vi "Apply Lowpass Filter.vi"(6 "state info in":T2 {"y(n-2) state" format="%.2f"; "x(n-2) state" format="%.2f"; "y(n-1) state" format="%.2f"; "x(n-1) state" format="%.2f"}, 7 "reset":bool=TRUE, 9 "filter coefficients":cluster{"beta":dbl, "gamma":dbl, "alpha":dbl} {"alpha" format="%.2f"; "gamma" format="%.2f"; "beta" format="%.2f"}, 10 "Conversion Op":T1, 11 "Input stream":waveform(sgl)={"t0"=timestamp(0 s since 1904-01-01), "dt"=0.0, "Y"=[]}) -> (3 "filtered signal":waveform(sgl), 4 "state info out":T2 {"y(n-2) state" format="%.2f"; "x(n-2) state" format="%.2f"; "y(n-1) state" format="%.2f"; "x(n-1) state" format="%.2f"})   [LabVIEW 2017, in "VibrationAnalysisFunctions.lvlib"]
uses:
  <vilib>/addons/InsightCM/Utilities/Analysis/Vibration/VibrationAnalysisFunctions.lvlib
  <vilib>/addons/InsightCM/Utilities/Analysis/Shared/controls/ConversionOp.ctl
  <vilib>/addons/InsightCM/Utilities/Analysis/Shared/AnalysisHelper.lvlib
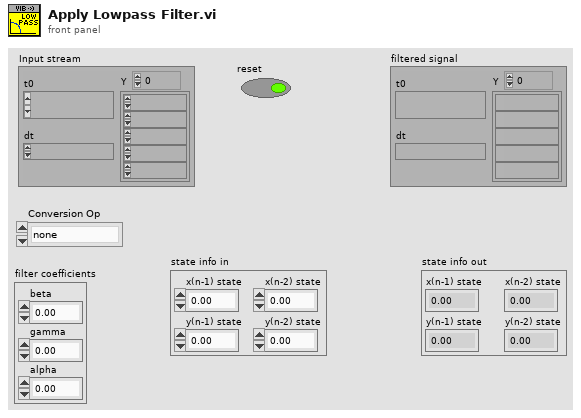
[diagram p1: front panel]
types:
  T1 = typedef "AnalysisHelper.lvlib/ConversionOp.ctl" = enum16{"none", "singleInt", "doubleInt", "singleDiff", "doubleDiff"}
  T2 = cluster{"x(n-1) state":dbl, "y(n-1) state":dbl, "x(n-2) state":dbl, "y(n-2) state":dbl}
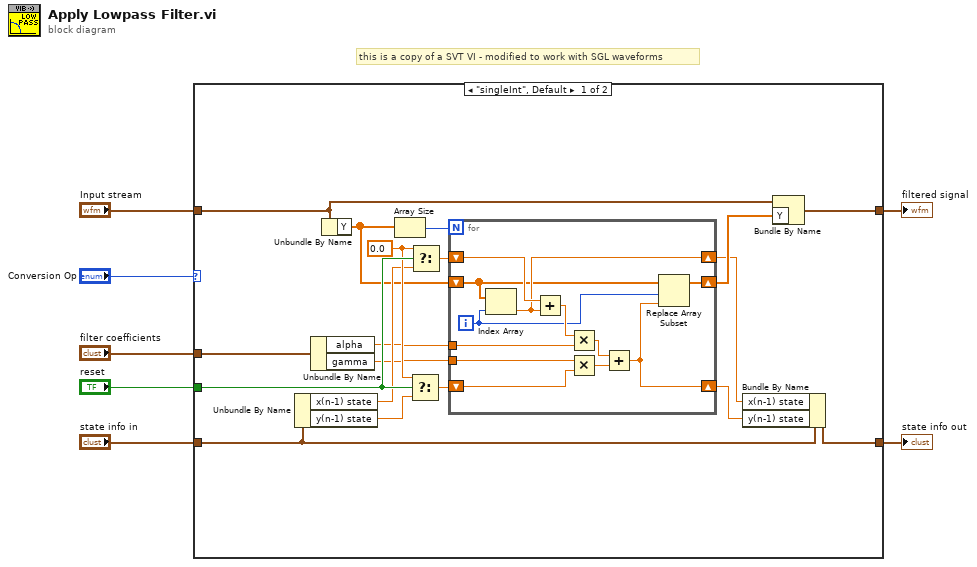
[diagram p0: block diagram]
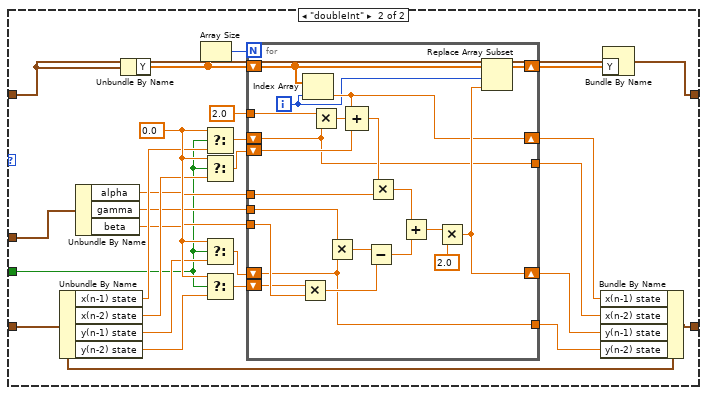
[diagram p2: hidden frame]
diagram:
  # "this is a copy of a SVT VI - modified to work with SGL waveforms"
  n1 = case shown="\"singleInt\", Default" "Conversion Op" {
    tunnel: "Input stream" -> [w24 w39]
    tunnel: "reset" -> [w23 w41]
    tunnel: "state info in" -> [w22 w42]
    tunnel: "filter coefficients" -> [w14 w40]
    tunnel: [w9 w43] -> w3
    tunnel: [w8 w38] -> w2
    frame "singleInt", Default {
      w17 = 0.0 ("Element Data")
      n2 = Unbundle By Name(w22) -> ("x(n-1) state"=w15:dbl, "y(n-1) state"=w19:dbl)
      n3 = Unbundle By Name(w14) -> ("alpha"=w13:dbl, "gamma"=w12:dbl)
      n4 = Unbundle By Name(w24) -> ("Y"=w10:sgl[])
      n5 = Array Size(array=w10) -> (size(s)=w11:i32)
      n6 = Select(t=w17, s=w23, f=w19) -> (s? t:f=w16:dbl)
      n7 = Select(t=w17, s=w23, f=w15) -> (s? t:f=w18:dbl)
      n8 = for {
        N: w11 -> [_]
        shift-right: [w30] -> w20
        shift-left: w18 -> [w37]
        tunnel: w13 -> [w31]
        shift-right: [w27] -> w21
        shift-left: w16 -> [w33]
        tunnel: w12 -> [w35]
        shift-right: [w28] -> w25
        shift-left: w10 -> [w29]
        i -> [w26]
        n9 = Index Array(array=w29, index=w26) -> (element=w30:sgl)
        n10 = Add(x=w37, y=w30) -> (x+y=w36:dbl)
        n11 = Multiply(x=w36, y=w31) -> (x*y=w32:dbl)
        n12 = Multiply(x=w35, y=w33) -> (x*y=w34:dbl)
        n13 = Add(x=w32, y=w34) -> (x+y=w27:dbl)
        n14 = Replace Array Subset(array=w29, new element=w27, index=w26) -> (w28:sgl[])
      }
      n15 = Bundle By Name(cluster=w22, "x(n-1) state"=w20, "y(n-1) state"=w21) -> (w9:T2)
      n16 = Bundle By Name(cluster=w24, "Y"=w25) -> (w8:waveform(sgl))
    }
    frame "doubleInt" {
      w63 = 0.0 ("x")
      n17 = Unbundle By Name(w42) -> ("x(n-1) state"=w52:dbl, "x(n-2) state"=w51:dbl, "y(n-1) state"=w61:dbl, "y(n-2) state"=w50:dbl)
      n18 = Unbundle By Name(w40) -> ("alpha"=w46:dbl, "gamma"=w47:dbl, "beta"=w48:dbl)
      n19 = Unbundle By Name(w39) -> ("Y"=w44:sgl[])
      n20 = Array Size(array=w44) -> (size(s)=w45:i32)
      n21 = Select(t=w63, s=w41, f=w52) -> (s? t:f=w55:dbl)
      n22 = Select(t=w63, s=w41, f=w51) -> (s? t:f=w54:dbl)
      n23 = Select(t=w63, s=w41, f=w61) -> (s? t:f=w56:dbl)
      n24 = Select(t=w63, s=w41, f=w50) -> (s? t:f=w53:dbl)
      n25 = for {
        N: w45 -> [_]
        shift-right: [w67] -> w60
        shift-left: w55 -> [w68]
        shift-left: w54 -> [w72]
        tunnel: 2.0 ("x") -> [w84]
        tunnel: w46 -> [w81]
        shift-right: [w73] -> w49
        shift-left: w56 -> [w71]
        shift-left: w53 -> [w70]
        tunnel: w47 -> [w69]
        tunnel: w48 -> [w77]
        tunnel: [w68] -> w59
        tunnel: [w71] -> w58
        shift-right: [w66] -> w62
        shift-left: w44 -> [w64]
        i -> [w65]
        n26 = Multiply(x=w70, y=w77) -> (x*y=w76:dbl)
        n27 = Index Array(array=w64, index=w65) -> (element=w67:sgl)
        n28 = Multiply(x=w84, y=w68) -> (x*y=w83:dbl)
        n29 = Multiply(x=w69, y=w71) -> (x*y=w79:dbl)
        n30 = Compound Arithmetic op=ADD(w67, w83, w72) -> (w82:dbl)
        n31 = Subtract(x=w79, y=w76) -> (x-y=w78:dbl)
        n32 = Multiply(x=w82, y=w81) -> (x*y=w80:dbl)
        n33 = Add(x=w80, y=w78) -> (x+y=w75:dbl)
        n34 = Multiply(x=w75, y=2.0) -> (x*y=w73:dbl)
        n35 = Replace Array Subset(array=w64, new element=w73, index=w65) -> (w66:sgl[])
      }
      n36 = Bundle By Name(cluster=w42, "x(n-1) state"=w60, "x(n-2) state"=w59, "y(n-1) state"=w49, "y(n-2) state"=w58) -> (w43:T2)
      n37 = Bundle By Name(cluster=w39, "Y"=w62) -> (w38:waveform(sgl))
    }
  }
  "filtered signal" <- w2
  "state info out" <- w3
